vi "Command Shoot.vi"(2 "All Robot Commands In":T5, 3 "Startup":bool, 4 "String Parameter":string, 5 "Ball Detection Time":dbl, 6 "Timeout":dbl, 7 "Time to Run":dbl) -> (0 "All Robot Commands Out":T5, 1 "Completed":bool)   [LabVIEW 2016]
uses:
  Subsystems/Drive and Climb SS/Drive + Climb Commands 2017.ctl
  Subsystems/Gear Delivery SS/Gear Delivery Commands.ctl
  Subsystems/Conveyor and Shooter SS/Conveyor and Shooter Commands.ctl
  Subsystems/Ball Intake SS/Ball Intake Commands.ctl
  Command Execution State.ctl
  Global Variables/Robot Status.vi
  Global Variables/Refnum Names.vi
panel:
  # "Sample robot\ncontrol output.\nReplace with \nactual teleop \ncontrol signal \nstructure."
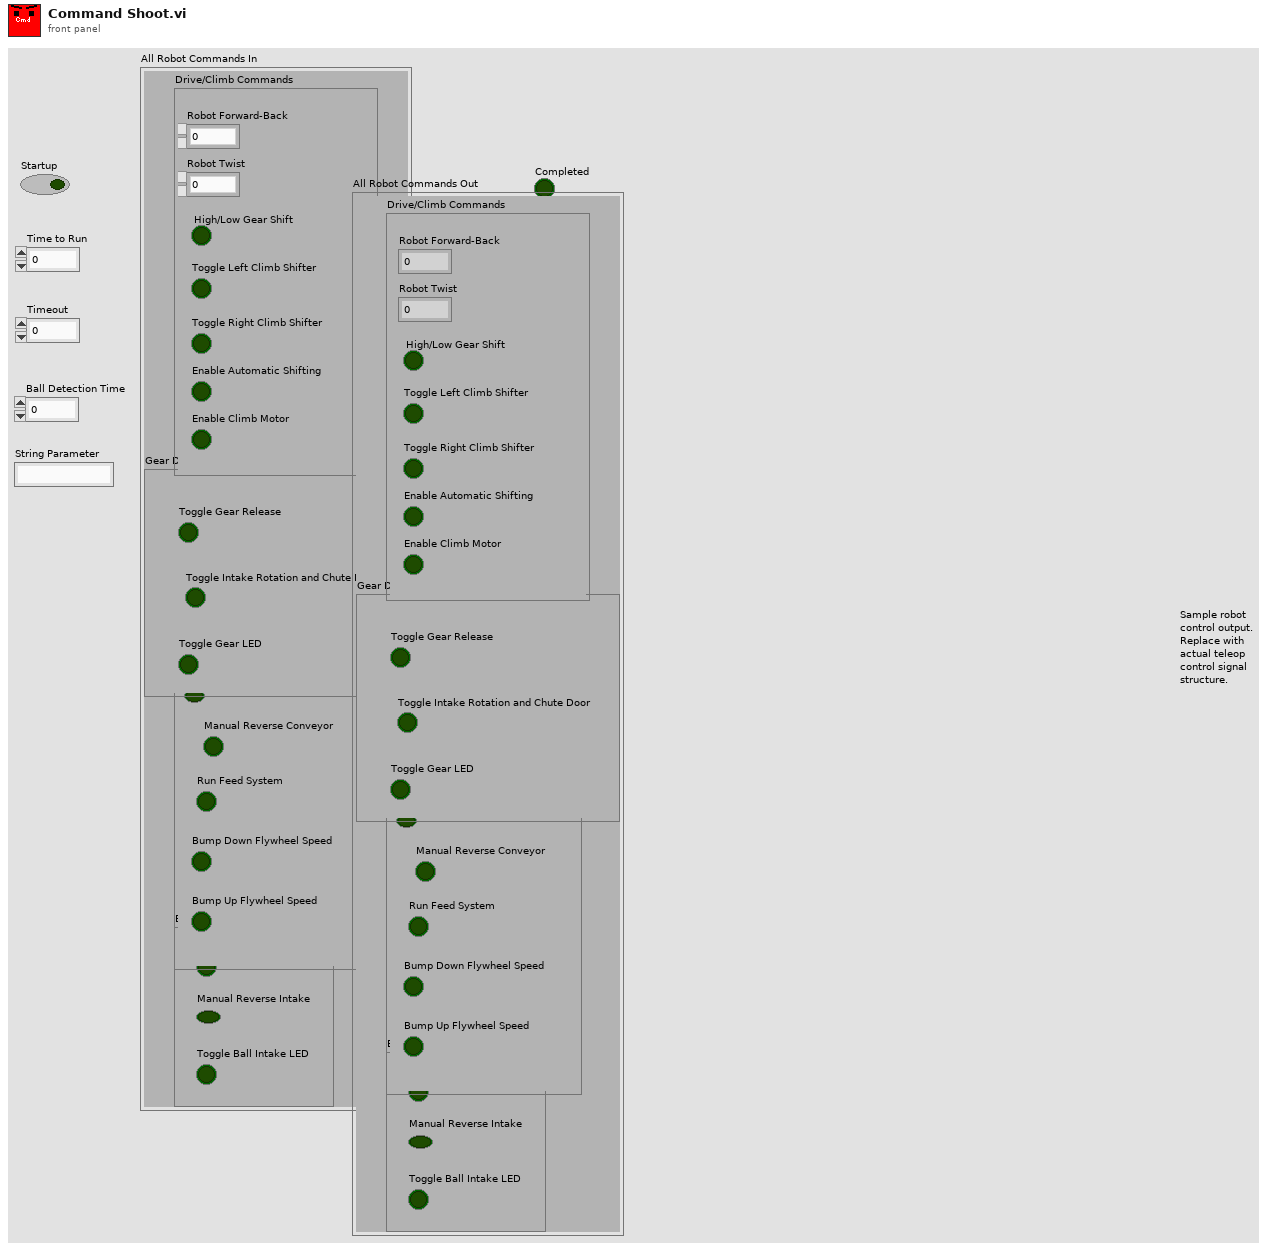
[diagram p1: front panel]
types:
  T1 = typedef "Drive + Climb Commands 2017.ctl" = cluster{"Robot Forward-Back":dbl, "Robot Twist":dbl, "High/Low Gear Shift":bool, "Toggle Left Climb Shifter":bool, "Toggle Right Climb Shifter":bool, "Enable Automatic Shifting":bool, "Enable Climb Motor ":bool}
  T2 = typedef "Gear Delivery Commands.ctl" = cluster{"Toggle Gear Release":bool, "Toggle Intake Rotation and Chute Door":bool, "Toggle Gear LED":bool}
  T3 = typedef "Conveyor and Shooter Commands.ctl" = cluster{"Toggle Shooter":bool, "Manual Reverse Conveyor":bool, "Run Feed System":bool, "Bump Down Flywheel Speed":bool, "Bump Up Flywheel Speed":bool}
  T4 = typedef "Ball Intake Commands.ctl" = cluster{"Toggle Ball Intake":bool, "Manual Reverse Intake":bool, "Toggle Ball Intake LED":bool}
  T5 = cluster{"Drive/Climb Commands":T1, "Gear Delivery Commands":T2, "Shooter and Conveyor Commands":T3, "Ball Intake Commands":T4}
  T6 = typedef "Command Execution State.ctl" = enum16{"Initialize", "Execute", "Finish"}
  T7 = typedef "WPI_DigitalInputDevRef.ctl" = cluster{"DevStatus":errorcluster, "DIO Channel":T8}
  T8 = typedef "FPGA_DIOChannel.ctl" = enum8{"DIO 0", "DIO 1", "DIO 2", "DIO 3", "DIO 4", "DIO 5", "DIO 6", "DIO 7", "DIO 8", "DIO 9", "DIO MXP 0", "DIO MXP 1", "DIO MXP 2", "DIO MXP 3", "DIO MXP 4", "DIO MXP 5", "DIO MXP 6", "DIO MXP 7", "DIO MXP 8", "DIO MXP 9", "DIO MXP 10", "DIO MXP 11", "DIO MXP 12", "DIO MXP 13", "DIO MXP 14", "DIO MXP 15", "SPI Port CS1", "SPI Port CS2", "SPI Port CS3", "SPI Port MISO", "SPI Port MOSI", "Invalid"}
  T9 = typedef "WPI_MotorControlDeviceRef.ctl" = cluster{"DeviceStatus":errorcluster, "Type":T10, "PWM":cluster{"PWM Channel":T11, "DeadBand":T12}, "CAN":cluster{"Device Number":u8, "SetOutput VI Ref":variant, "GetOutput VI Ref":variant, "Enable VI Ref":variant, "Disable VI Ref":variant, "Data":variant}, "Invert":bool}
  T10 = typedef "WPI_MotorControlType.ctl" = enum16{"PWM", "CAN"}
  T11 = typedef "FPGA_DIOPWMChannel.ctl" = enum8{"PWM 0", "PWM 1", "PWM 2", "PWM 3", "PWM 4", "PWM 5", "PWM 6", "PWM 7", "PWM 8", "PWM 9", "PWM MXP 0", "PWM MXP 1", "PWM MXP 2", "PWM MXP 3", "PWM MXP 4", "PWM MXP 5", "PWM MXP 6", "PWM MXP 7", "PWM MXP 8", "PWM MXP 9", "Invalid"}
  T12 = typedef "WPI_PWMDeadband.ctl" = cluster{"Name":string, "maxPositivePwm":i32, "minPositivePwm":i32, "centerPwm":i32, "maxNegativePwm":i32, "minNegativePwm":i32, "angularRange":u16}
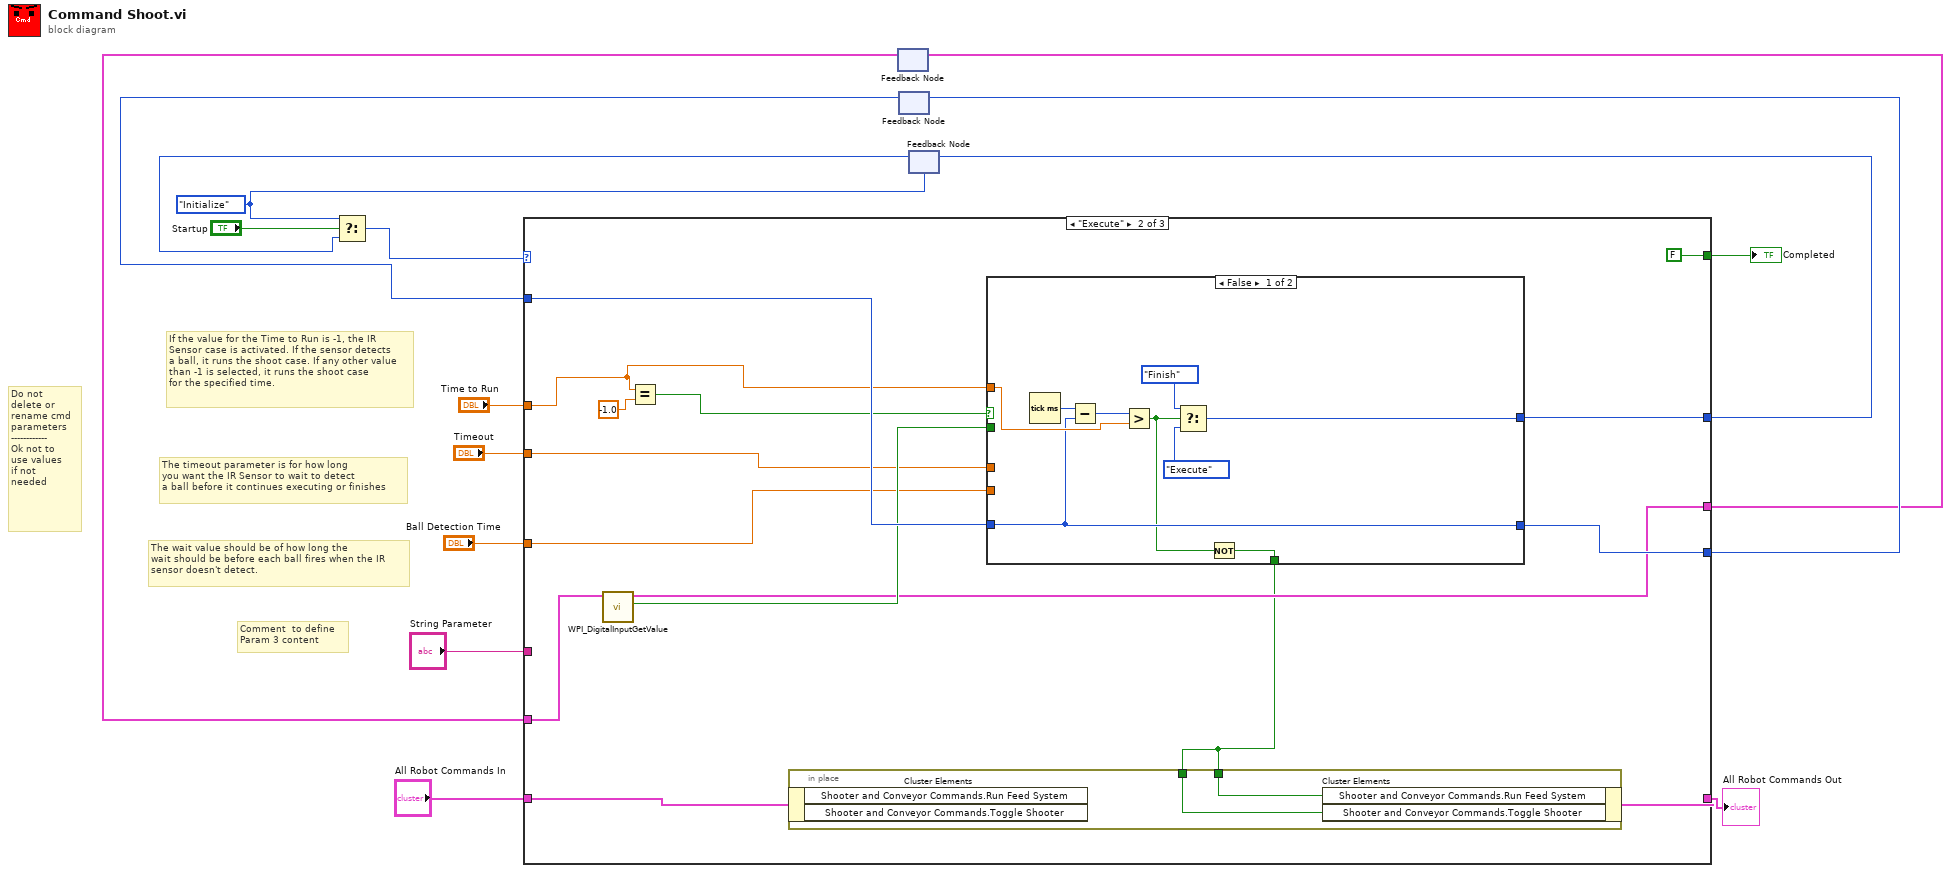
[diagram p0: block diagram]
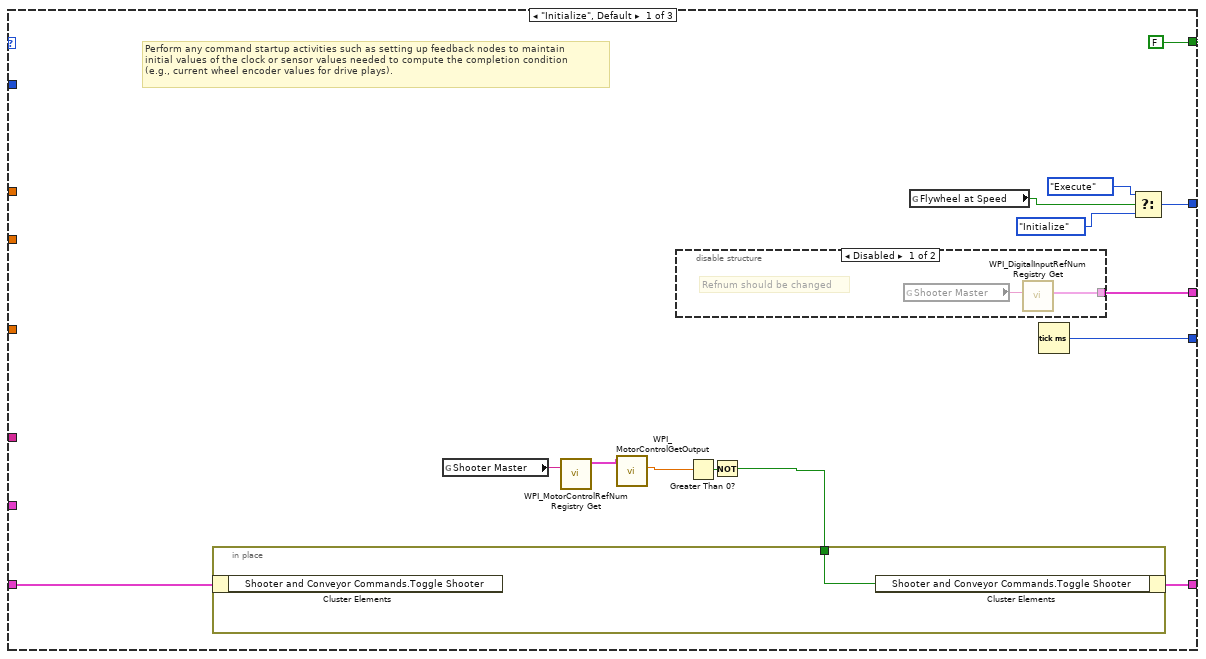
[diagram p2: hidden frame]
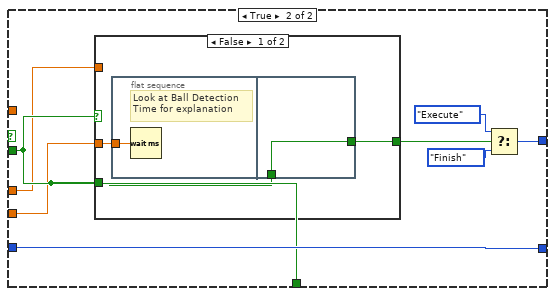
[diagram p4: hidden frame]
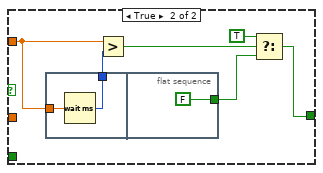
[diagram p5: hidden frame]
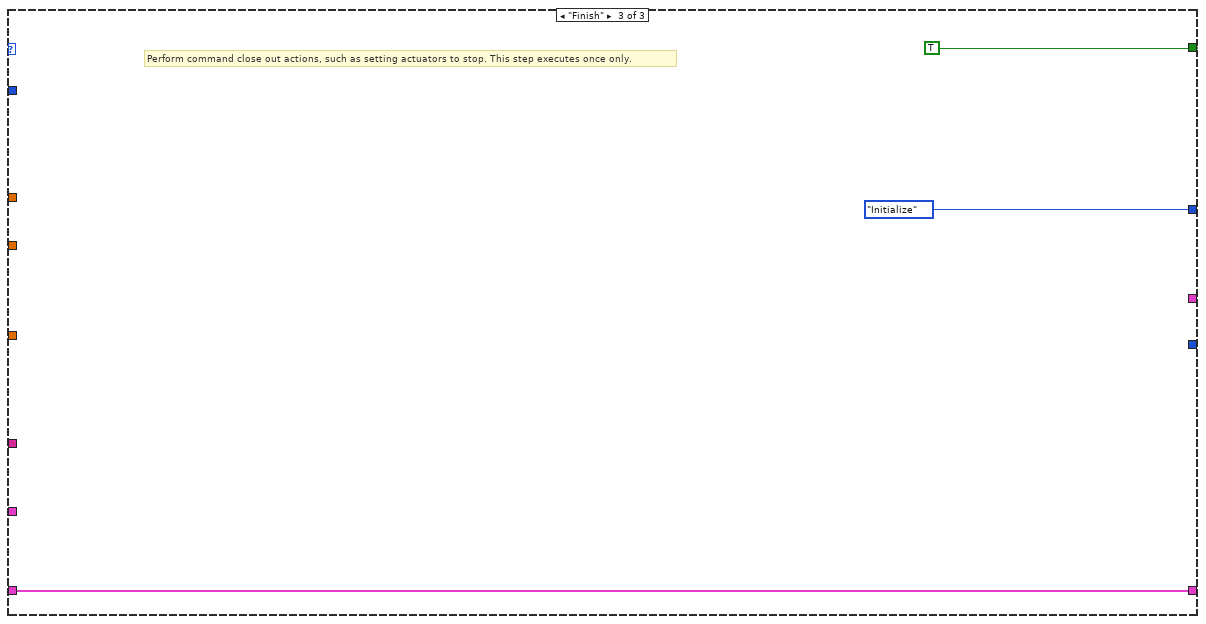
[diagram p6: hidden frame]
diagram:
  w11 = Command_Execution_State."Initialize" ("Play State")
  # "The wait value should be of how long the \nwait should be before each ball fires when the IR \nsensor doesn't detect."
  # "If the value for the Time to Run is -1, the IR \nSensor case is activated. If the sensor detects\na ball, it runs the shoot case. If any other value\nthan -1 is selected, it runs the shoot case\nfor the specified time."
  # "Comment  to define\nParam 3 content"
  # "Do not \ndelete or\nrename cmd\nparameters\n------------\nOk not to \nuse values\nif not \nneeded"
  # "The timeout parameter is for how long\nyou want the IR Sensor to wait to detect \na ball before it continues executing or finishes"
  n1 = feedback #1() -> (w3:T7)  [unwired: 1 in]
  n2 = feedback #2() -> (w5:u32)  [unwired: 1 in]
  n3 = feedback #3(w11) -> (w12:T6)
  n4 = Select(t=w11, s="Startup", f=w12) -> (s? t:f=w16:T6)
  n5 = case shown="\"Execute\"" w16 {
    tunnel: [FALSE FALSE TRUE] -> w14
    tunnel: [w25 w47 Command_Execution_State."Initialize" ("f")] -> w13
    tunnel: "Time to Run" -> [_ w36 _]
    tunnel: "Timeout" -> [_ w37 _]
    tunnel: [w23 w39 w82] -> w1
    tunnel: "All Robot Commands In" -> [w19 w43 w82]
    tunnel: "Ball Detection Time" -> [_ w40 _]
    tunnel: "String Parameter" -> [_ _ _]
    tunnel: [w30 w38 _] -> w6
    tunnel: w5 -> [_ w46 _]
    tunnel: [w20 w35 _] -> w4
    tunnel: w3 -> [_ w44 _]
    frame "Initialize", Default {
      # "Perform any command startup activities such as setting up feedback nodes to maintain \ninitial values of the clock or sensor values needed to compute the completion condition\n(e.g., current wheel encoder values for drive plays)."
      n6 = global read "Refnum Names.vi" "Shooter Master"() -> (w22:string)
      n7 = call <vilib>:"WPI_MotorControlRefNum Registry Get.vi"("refnum name"=w22) -> ("MotorControlDevRef"=w21:T9)  [unwired: 9 in, 1 out]
      n8 = call <vilib>:"WPI_MotorControlGetOutput.vi"("MotorControlDevRef"=w21) -> ("Output"=w24:dbl)  [unwired: 8 in, 2 out]
      n9 = disable-structure shown="Disabled" {
        disable-tunnel: [w31 _] -> w20
        frame Disabled {
          # "Refnum should be changed"
          n10 = global read "Refnum Names.vi" "Shooter Master"() -> (w32:string)
          n11 = call <vilib>:"WPI_DigitalInputRefNum Registry Get.vi"("refnum name"=w32) -> ("DigitalInputDevRef"=w31:T7)  [unwired: 9 in, 1 out]
        }
        frame Enabled {
        }
      }
      n12 = Greater Than 0?(x=w24) -> (x > 0?=w18:bool)
      n13 = Not(x=w18) -> (.not. x?=w17:bool)
      n14 = in-place {
        in-place-border: w17 -> [w33]
        n15 = in-place-cluster #4(w19) -> ()  [unwired: 1 out]
        n16 = in-place-cluster #4("Shooter and Conveyor Commands.Toggle Shooter"=w33) -> (w23:T5)
      }
      n17 = global read "Robot Status.vi" "Flywheel at Speed"() -> (w29:bool)
      n18 = Tick Count (ms)() -> (millisecond timer value=w30:u32)
      n19 = Select(t=Command_Execution_State."Execute" ("Play State"), s=w29, f=Command_Execution_State."Initialize") -> (s? t:f=w25:T6)
    }
    frame "Execute" {
      n20 = call <vilib>:"WPI_DigitalInputGetValue.vi"("DigitalInputDevRef"=w44) -> ("Value"=w42:bool, "DigitalInputDevRef"=w35:T7)  [unwired: 8 in, 1 out]
      n21 = Equal?(x=w36, y=-1.0) -> (x = y?=w41:bool)
      n22 = case shown="False" w41 {
        tunnel: [w56 w61] -> w47
        tunnel: w36 -> [w52 _]
        tunnel: w46 -> [w51 w65]
        tunnel: [w51 w65] -> w38
        tunnel: w42 -> [_ w64]
        tunnel: [w49 w64] -> w34
        tunnel: w37 -> [_ w59]
        tunnel: w40 -> [_ w58]
        frame False {
          n23 = Tick Count (ms)() -> (millisecond timer value=w54:u32)
          n24 = Subtract(x=w54, y=w51) -> (x-y=w53:u32)
          n25 = Greater?(x=w53, y=w52) -> (0:w50:bool)
          n26 = Select(t=Command_Execution_State."Finish" ("Play State"), s=w50, f=Command_Execution_State."Execute") -> (s? t:f=w56:T6)
          n27 = Not(x=w50) -> (.not. x?=w49:bool)
        }
        frame True {
          n28 = case shown="False" w64 {
            tunnel: [w66 w71] -> w60
            tunnel: w64 -> [w68 _]
            tunnel: w59 -> [_ w75]
            tunnel: w58 -> [w67 _]
            frame False {
              n29 = flat-sequence {
                tunnel: w67 -> [w69]
                tunnel: [w70] -> w66
                tunnel: w68 -> [w70]
                frame #0 {
                  # "Look at Ball Detection \nTime for explanation"
                  n30 = Wait (ms)(milliseconds to wait=w69) -> ()  [unwired: 1 out]
                }
                frame #1 {
                }
              }
            }
            frame True {
              n31 = flat-sequence {
                tunnel: w75 -> [w78]
                tunnel: [w77] -> w72
                tunnel: [FALSE] -> w73
                frame #0 {
                  n32 = Wait (ms)(milliseconds to wait=w78) -> (millisecond timer value=w77:u32)
                }
                frame #1 {
                }
              }
              n33 = Greater?(x=w75, y=w72) -> (0:w74:bool)
              n34 = Select(t=TRUE, s=w74, f=w73) -> (s? t:f=w71:bool)
            }
          }
          n35 = Select(t=Command_Execution_State."Execute" ("Play State"), s=w60, f=Command_Execution_State."Finish") -> (s? t:f=w61:T6)
        }
      }
      n36 = in-place {
        in-place-border: w34 -> [w80]
        in-place-border: w34 -> [w81]
        n37 = in-place-cluster #5(w43) -> ()  [unwired: 2 out]
        n38 = in-place-cluster #5("Shooter and Conveyor Commands.Run Feed System"=w80, "Shooter and Conveyor Commands.Toggle Shooter"=w81) -> (w39:T5)
      }
    }
    frame "Finish" {
      # "Perform command close out actions, such as setting actuators to stop. This step executes once only."
    }
  }
  "Completed" <- w14
  "All Robot Commands Out" <- w1
  n39 = feedback-in #1(w4) -> ()
  n40 = feedback-in #2(w6) -> ()
  n41 = feedback-in #3(w13) -> ()
